vi "생산자소비자(상태머신).vi"() -> ()   [LabVIEW 2014]
uses:
  Status.ctl
  <vilib>/Analysis/NI_AALBase.lvlib
panel:
  in  "긴급":bool
  in  "삼각파":bool
  out "웨이브폼 그래프":dbl[](graph)
  in  "사인파":bool
  in  "정지":bool
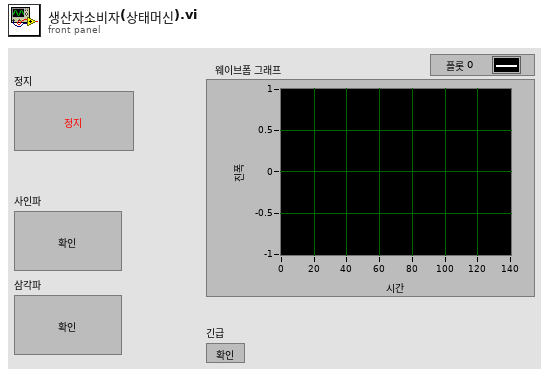
[diagram p1: front panel]
types:
  T1 = typedef "Status.ctl" = enum16{"Idle", "초기화", "정지", "Task1", "Task2", "기다림"}
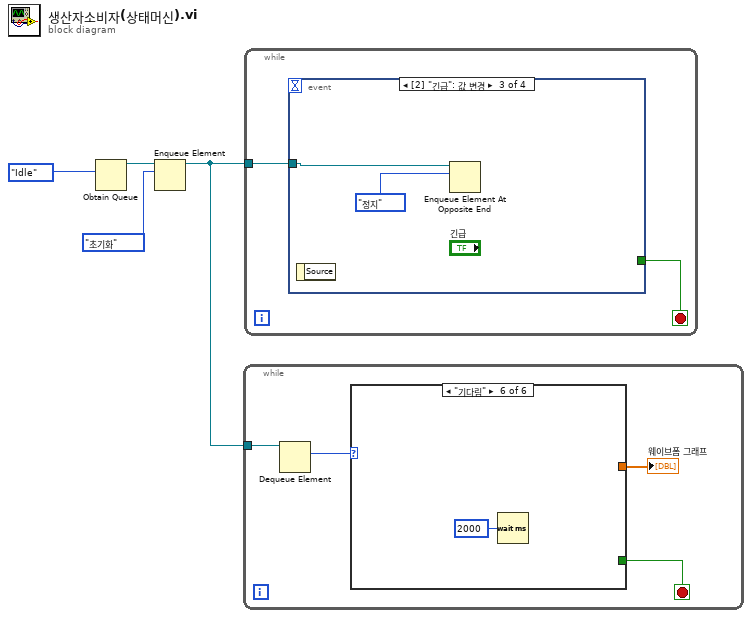
[diagram p0: block diagram]
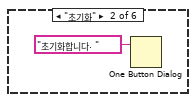
[diagram p3: hidden frame]
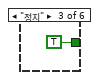
[diagram p4: hidden frame]
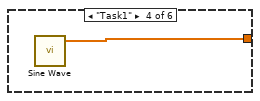
[diagram p5: hidden frame]
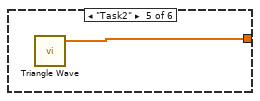
[diagram p6: hidden frame]
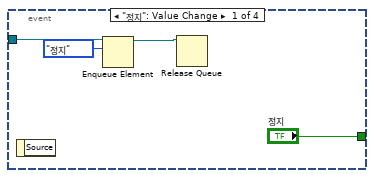
[diagram p7: hidden frame]
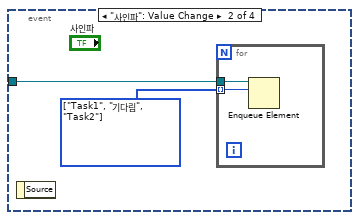
[diagram p8: hidden frame]
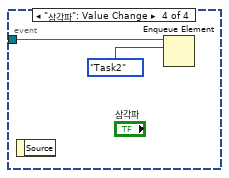
[diagram p9: hidden frame]
diagram:
  n1 = Obtain Queue(element data type=Status."Idle" ("상태")) -> (queue out=w4:refnum<queue>)  [unwired: 4 in, 2 out]
  n2 = Enqueue Element(queue=w4, element=Status."초기화" ("원소")) -> (queue out=w3:refnum<queue>)  [unwired: 2 in, 2 out]
  n3 = while {
    tunnel: w3 -> [w8]
    stop <- w6 stop-if-true
    n4 = Dequeue Element(queue=w8) -> (element=w7:T1)  [unwired: 2 in, 3 out]
    n5 = case shown="\"기다림\"" w7 {
      tunnel: [_ _ TRUE _ _ _] -> w6
      tunnel: [_ _ _ w11 w12 _] -> w5
      frame "Idle", Default {
      }
      frame "초기화" {
        n6 = One Button Dialog(message="초기화합니다. " ("메시지")) -> ()  [unwired: 1 in, 1 out]
      }
      frame "정지" {
      }
      frame "Task1" {
        n7 = call <vilib>:"Sine Wave.vi"() -> ("sine wave"=w11:dbl[])  [unwired: 5 in, 2 out]
      }
      frame "Task2" {
        n8 = call <vilib>:"Triangle Wave.vi"() -> ("triangle wave"=w12:dbl[])  [unwired: 5 in, 2 out]
      }
      frame "기다림" {
        n9 = Wait (ms)(milliseconds to wait=u32 2000 ("대기 시간(ms)")) -> ()  [unwired: 1 out]
      }
    }
    "웨이브폼 그래프" <- w5
  }
  n10 = while {
    tunnel: w3 -> [w15]
    stop <- w14 stop-if-true
    n11 = event shown="[2] \"긴급\": 값 변경" {
      selector: _ -> [_ _ _ _]
      dyn-events: _ -> [_ _ _ _]
      timeout: _ -> [_ _ _ _]
      tunnel: w15 -> [w18 w21 w25 w27]
      tunnel: ["정지" _ _ _] -> w14
      event "정지": Value Change {
        n12 = event-data() -> ()  [unwired: 1 in, 1 out]
        n13 = Enqueue Element(queue=w18, element=Status."정지" ("원소")) -> (queue out=w17:refnum<queue>)  [unwired: 2 in, 2 out]
        n14 = Release Queue(queue=w17) -> ()  [unwired: 2 in, 3 out]
      }
      event "사인파": Value Change {
        w20 = T1[] [enum."Task1", enum."기다림", enum."Task2"] items=["Idle", "초기화", "정지", "Task1", "Task2", "기다림"]
        n15 = event-data() -> ()  [unwired: 1 in, 1 out]
        n16 = for {
          tunnel: w21 -> [w23]
          tunnel: w20 -> [w22] mode=indexing
          n17 = Enqueue Element(queue=w23, element=w22) -> ()  [unwired: 2 in, 3 out]
        }
      }
      event "긴급": Value Change {
        n18 = event-data() -> ()  [unwired: 1 in, 1 out]
        n19 = Enqueue Element At Opposite End(queue=w25, element=Status."정지" ("원소")) -> ()  [unwired: 2 in, 3 out]
      }
      event "삼각파": Value Change {
        n20 = event-data() -> ()  [unwired: 1 in, 1 out]
        n21 = Enqueue Element(queue=w27, element=Status."Task2" ("상태")) -> ()  [unwired: 2 in, 3 out]
      }
    }
  }
